vi "Database.Main-Init.vi"(8 "error in":errorcluster) -> (0 "error out":errorcluster)   [LabVIEW 2016]
uses:
  Database.Main.Action.ctl
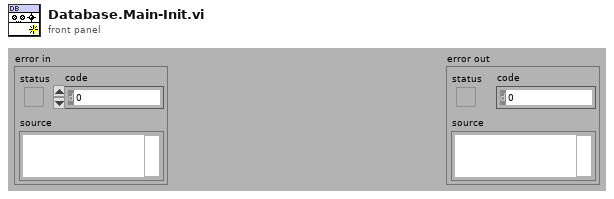
[diagram p1: front panel]
types:
  T1 = typedef "Database.Main.Action.ctl" = enum32{"idle", "constructor", "destructor", "--- DB ---", "Init", "Setup", "Select.Variant", "File.Export", "UpdateVariantFiles", "CheckStatus"}
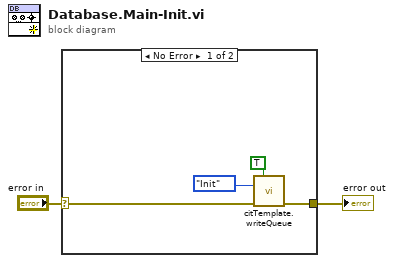
[diagram p0: block diagram]
diagram:
  n1 = case shown="No Error" "error in" {
    selector: "error in" -> [w5 w7]
    tunnel: [w6 w7] -> w1
    frame No Error {
      n2 = call "citTemplate.writeQueue.vi"("High priority (F)"=TRUE, "event in (if not connected:all statemachine with data event)"=Database.Main.Action."Init" ("Action"), "error in (no error)"=w5) -> ("error out"=w6:errorcluster)  [unwired: 12 in]
    }
    frame Error {
    }
  }
  "error out" <- w1
